vi "Get Gplugin Data File.vi"(7 "error if not found":bool=TRUE, 8 "error in":errorcluster, 10 "library name":string, 11 "project ref":refnum<vi>) -> (0 "error out":errorcluster, 1 "found":bool, 2 "Document item":refnum<vi>, 3 "project ref out":refnum<vi>)   [LabVIEW 2021, in "InstrumentStudio Plug-In Editor.lvlib"]
uses:
  InstrumentStudio Plug-In Editor.lvlib
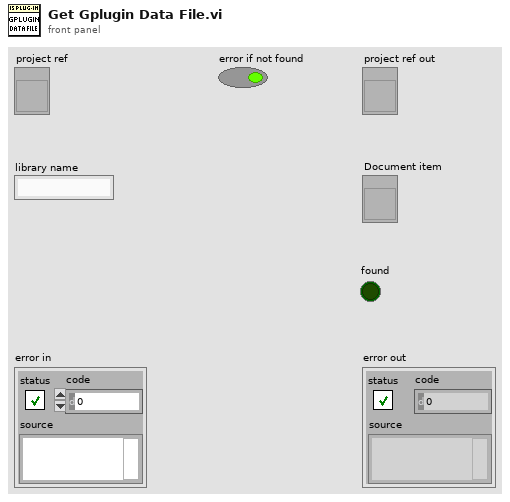
[diagram p1: front panel]
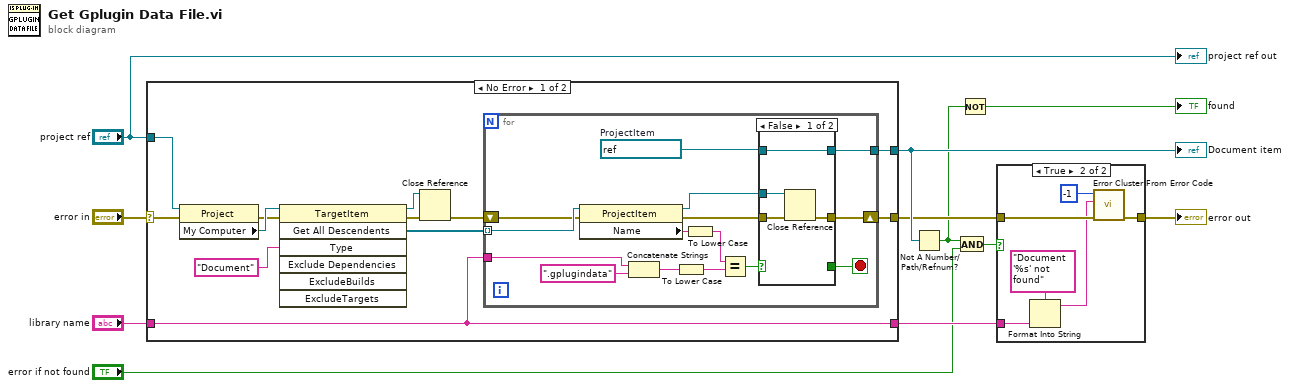
[diagram p0: block diagram]
diagram:
  n1 = case shown="No Error" "error in" {
    selector: "error in" -> [w19 w47]
    tunnel: "project ref" -> [w23 _]
    tunnel: "library name" -> [w13 w46]
    tunnel: [w18 w47] -> w6
    tunnel: [w14 _] -> w8
    tunnel: [w13 w46] -> w5
    frame No Error {
      n2 = property class="Project"(reference=w23, error in=w19) -> (error out=w21:errorcluster, "My Computer"=w22:refnum<vi>)  [unwired: 1 out]
      n3 = invoke class="TargetItem" method="Get All Descendents"(reference=w22, error in=w21, "Type"="Document") -> (reference out=w16:refnum<vi>, error out=w17:errorcluster, "All Descendents"=w20:refnum<vi>[])  [unwired: 4 in, 4 out]
      n4 = Close Reference(reference=w16, error in (no error)=w17) -> (error out=w15:errorcluster)
      n5 = for {
        tunnel: w20 -> [w38] mode=indexing
        tunnel: w13 -> [w37]
        shift-right: [w31] -> w18
        shift-left: w15 -> [w35]
        tunnel: [w30] -> w14
        stop <- w25 stop-if-true
        w24 = refnum<vi> refnum  # ProjectItem
        n6 = property class="ProjectItem"(reference=w38, error in=w35) -> (reference out=w33:refnum<vi>, error out=w34:errorcluster, "Name"=w27:string)
        n7 = Concatenate Strings(w37, ".gplugindata" ("string")) -> (w29:string)
        n8 = To Lower Case(string=w29) -> (all lower case string=w28:string)
        n9 = To Lower Case(string=w27) -> (all lower case string=w26:string)
        n10 = Equal?(x=w26, y=w28) -> (x = y?=w32:bool)
        n11 = case shown="False" w32 {
          selector: w32 -> [_ w43]
          tunnel: w34 -> [w42 w45]
          tunnel: w33 -> [w39 w44]
          tunnel: [w41 w45] -> w31
          tunnel: [w40 w44] -> w30
          tunnel: w24 -> [w40 _]
          tunnel: [_ w43] -> w25
          frame False {
            n12 = Close Reference(reference=w39, error in (no error)=w42) -> (error out=w41:errorcluster)
          }
          frame True {
          }
        }
      }
    }
    frame Error {
    }
  }
  "Document item" <- w8
  n13 = Not A Number/Path/Refnum?(number/path/refnum=w8) -> (NaN/Path/Refnum?=w2:bool)
  n14 = And(x=w2, y="error if not found") -> (x .and. y?=w4:bool)
  n15 = Not(x=w2) -> (.not. x?=→"found":bool)
  n16 = case shown="True" w4 {
    tunnel: [w48 w54] -> w7
    tunnel: w6 -> [w48 w53]
    tunnel: w5 -> [_ w49]
    frame False {
    }
    frame True {
      n17 = Format Into String(format string="Document '%s' not found" ("initial string"), w49) -> (resulting string=w50:string)  [unwired: 2 in, 1 out]
      n18 = call <vilib>:"Error Cluster From Error Code.vi"("error in (no error)"=w53, "error message (\"\")"=w50, "error code (0)"=-1) -> ("error out"=w54:errorcluster)  [unwired: 6 in]
    }
  }
  "error out" <- w7
  "project ref out" <- "project ref"
